vi "Write EvtReportArray.vi"(8 "error in (no error)":errorcluster, 10 "clEvtReportArray":T1 {"Synx" format="%#_4g"}, 11 "EventPluginBaseClass in":refnum<class "EventPluginBaseClass.lvclass">) -> (0 "error out":errorcluster, 3 "EventPluginBaseClass out":refnum<class "EventPluginBaseClass.lvclass">)   [LabVIEW 2017, in "EventPlugins.lvlib" / "EventPluginBaseClass.lvclass"]
uses:
  EventPluginBaseClass.lvclass
  TypeDefs/clEvtReportArray.ctl
  TypeDefs/clEvtReport.ctl
  EventPluginBaseClass.lvclass/EventPluginBaseClass.ctl
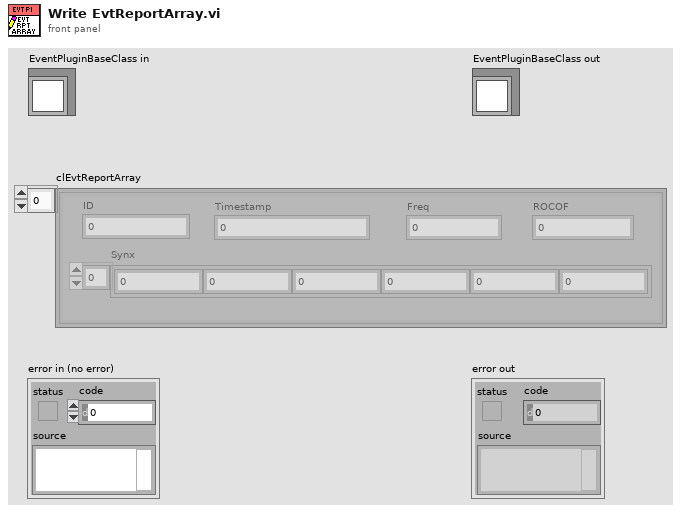
[diagram p1: front panel]
types:
  T1 = typedef "EventPlugins.lvlib/EventPluginBaseClass.lvclass/clEvtReportArray.ctl" = T2[]
  T2 = typedef "EventPlugins.lvlib/EventPluginBaseClass.lvclass/clEvtReport.ctl" = cluster{"Timestamp":dbl, "Synx":cdb[], "Freq":dbl, "ROCOF":dbl, "ID":i16}
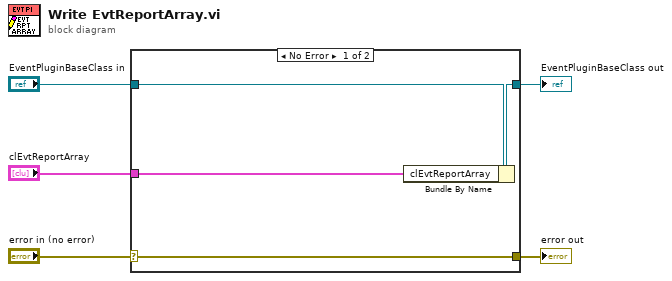
[diagram p0: block diagram]
diagram:
  n1 = case shown="No Error" "error in (no error)" {
    selector: "error in (no error)" -> [w9 w10]
    tunnel: [w9 w10] -> w4
    tunnel: [w7 w11] -> w2
    tunnel: "EventPluginBaseClass in" -> [w8 w11]
    tunnel: "clEvtReportArray" -> [w6 _]
    frame No Error {
      n2 = Bundle By Name(cluster=w8, "clEvtReportArray"=w6) -> (w7:refnum<class "EventPluginBaseClass.lvclass">)
    }
    frame Error {
    }
  }
  "error out" <- w4
  "EventPluginBaseClass out" <- w2
